vi "Node.Table.Find.vi"(8 "error in (no error)":errorcluster, 11 "Node":refnum<k24>) -> (0 "error out":errorcluster, 1 "Values":dbl[](array[numeric]), 2 "Names":string[](array[string]), 3 "Items":string[][](array[string]), 4 "Found?":bool)   [LabVIEW 2015, in "Workspace.Obejct.Radio.lvlib"]
uses:
  Workspace.Obejct.Radio.lvlib
  NationalInstruments.VeriStand.SystemStorage
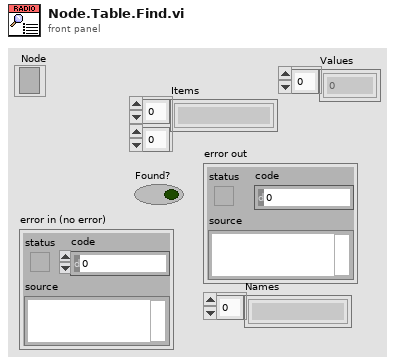
[diagram p1: front panel]
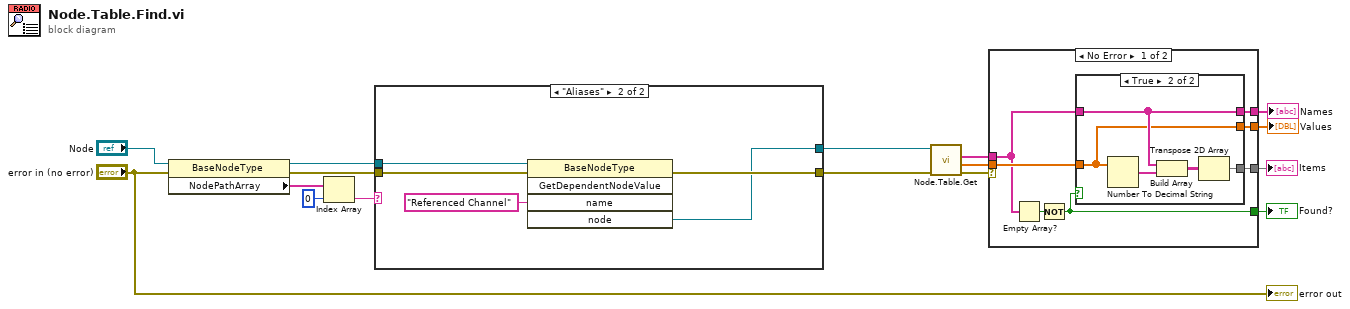
[diagram p0: block diagram]
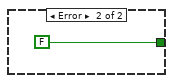
[diagram p4: hidden frame]
diagram:
  n1 = property class="BaseNodeType"(reference="Node", error in="error in (no error)") -> (reference out=w3:refnum<k24>, error out=w4:errorcluster, "NodePathArray"=w7:string[])
  n2 = Index Array(array=w7, index=0) -> (element=w5:string)
  n3 = case shown="\"Aliases\"" w5 {
    tunnel: w3 -> [w18 w23]
    tunnel: w4 -> [w17 w22]
    tunnel: [w18 w19] -> w2
    tunnel: [w17 w20] -> w1
    frame Default {
    }
    frame "Aliases" {
      n4 = invoke class="BaseNodeType" method="GetDependentNodeValue"(reference=w23, error in=w22, "name"="Referenced Channel") -> (error out=w20:errorcluster, "node"=w19:refnum<k24>)  [unwired: 2 in, 3 out]
    }
  }
  n5 = call "Node.Table.Get.vi"("error in (no error)"=w1, "Node"=w2) -> ("error out"=w10:errorcluster, "Values"=w12:dbl[], "Names"=w11:string[])  [unwired: 6 in, 1 out]
  n6 = case shown="No Error" w10 {
    tunnel: w11 -> [w28 _]
    tunnel: w12 -> [w30 _]
    tunnel: [w26 _] -> w16
    tunnel: [w27 FALSE] -> w15
    tunnel: [w25 _] -> w14
    tunnel: [w24 _] -> w13
    frame No Error {
      n7 = Empty Array?(array=w28) -> (empty?=w29:bool)
      n8 = Not(x=w29) -> (.not. x?=w27:bool)
      n9 = case shown="True" w27 {
        tunnel: w30 -> [_ w31]
        tunnel: w28 -> [_ w32]
        tunnel: [_ w33] -> w26
        tunnel: [_ w32] -> w25
        tunnel: [_ w31] -> w24
        frame False {
        }
        frame True {
          n10 = Number To Decimal String(number=w31) -> (decimal integer string=w35:string[])  [unwired: 1 in]
          n11 = Build Array(w32, w35) -> (w34:string[][])
          n12 = Transpose 2D Array(2D array=w34) -> (transposed array=w33:string[][])
        }
      }
    }
    frame Error {
    }
  }
  "Found?" <- w15
  "Items" <- w16
  "Names" <- w14
  "Values" <- w13
  "error out" <- "error in (no error)"
